vi "FGV SpecAn Model.vi"(4 "Action":T2, 5 "Error In":errorcluster, 8 "VISA In":refnum<visa-resource-name>) -> (0 "Error Out":errorcluster, 3 "SA Model":T1)   [LabVIEW 2015]
uses:
  Controls/FGV Action SpecAn Model.ctl
  Controls/SpecAn Model.ctl
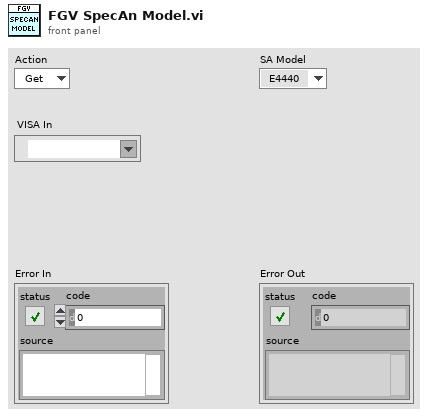
[diagram p1: front panel]
types:
  T1 = typedef "SpecAn Model.ctl" = enum16{"E4440", "N9030"}
  T2 = typedef "FGV Action SpecAn Model.ctl" = enum16{"Get", "Set"}
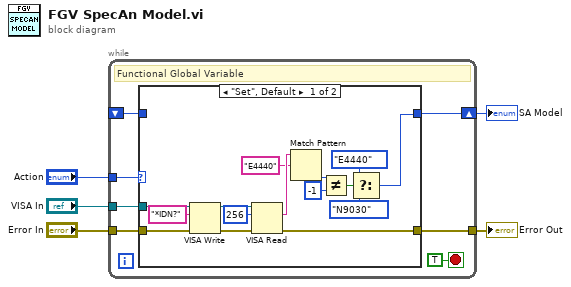
[diagram p0: block diagram]
diagram:
  n1 = while {
    shift-right: [w10] -> w1
    shift-left: _ -> [w9]
    tunnel: "Action" -> [w11]
    tunnel: "Error In" -> [w8]
    tunnel: [w7] -> w3
    tunnel: "VISA In" -> [w6]
    stop <- TRUE stop-if-true
    # "Functional Global Variable"
    n2 = case shown="\"Set\", Default" w11 {
      tunnel: [w13 w28] -> w10
      tunnel: w9 -> [_ w28]
      tunnel: w8 -> [w27 w29]
      tunnel: [w21 w29] -> w7
      tunnel: w6 -> [w26 _]
      frame "Set", Default {
        n3 = VISA Write(VISA resource name=w26, write buffer="*IDN?", error in (no error)=w27) -> (VISA resource name out=w23:refnum<visa-resource-name>, error out=w24:errorcluster)  [unwired: 1 out]
        n4 = VISA Read(VISA resource name=w23, byte count=u32 256, error in (no error)=w24) -> (read buffer=w20:string, error out=w21:errorcluster)  [unwired: 2 out]
        n5 = Match Pattern(string=w20, regular expression="E4440") -> (offset past match=w18:i32)  [unwired: 1 in, 3 out]
        n6 = Not Equal?(x=w18, y=-1) -> (x != y?=w16:bool)
        n7 = Select(t=SpecAn_Model."E4440" ("Model"), s=w16, f=SpecAn_Model."N9030" ("Model")) -> (s? t:f=w13:T1)
      }
      frame "Get" {
      }
    }
  }
  "Error Out" <- w3
  "SA Model" <- w1
